vi "Get Item by key.vi"(8 "error in (no error)":errorcluster caption="错误输入（无错误）", 10 "Key":variant, 11 "HashTable 输入":refnum<class "HashTable.lvclass"> caption="DNL_LabVIEW Object in") -> (0 "error out":errorcluster caption="错误输出", 2 "Value":variant, 3 "HashTable 输出":refnum<class "HashTable.lvclass"> caption="DNL_LabVIEW Object out")   [LabVIEW 2012, in "HashTable.lvclass"]
uses:
  HashTable.lvclass
  HashTable.lvclass/HashTable.ctl
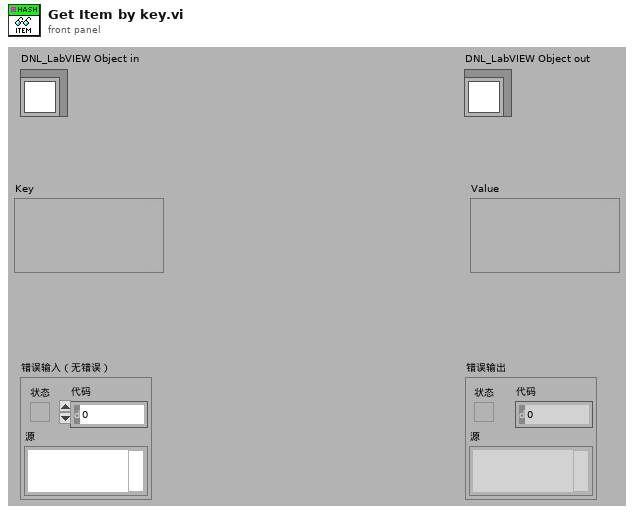
[diagram p1: front panel]
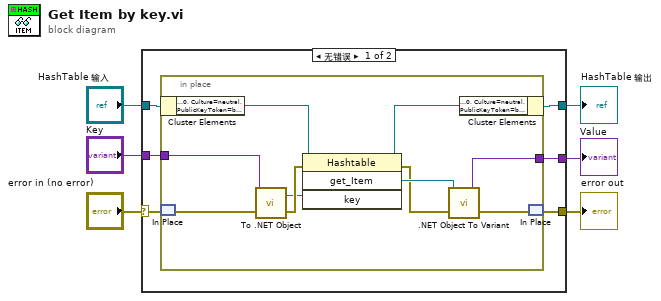
[diagram p0: block diagram]
diagram:
  n1 = case shown="无错误" "error in (no error)" {
    selector: "error in (no error)" -> [w10 w24]
    tunnel: [w7 w24] -> w5
    tunnel: [w11 w23] -> w3
    tunnel: "HashTable 输入" -> [w12 w23]
    tunnel: "Key" -> [w9 _]
    tunnel: [w8 _] -> w1
    frame No Error {
      n2 = in-place {
        in-place-border: w9 -> [w18]
        in-place-border: [w15] -> w8
        n3 = in-place-cluster #1(w12) -> ("HashTable"=w22:refnum<k24>)
        n4 = in-place-match #2(w10) -> (w20:errorcluster)
        n5 = call <vilib>:"To .NET Object.vi"("error in (no error)"=w20, "anything"=w18) -> ("error out"=w19:errorcluster, ".NET object"=w13:refnum<k24>)
        n6 = invoke class="Hashtable" method="get_Item"(reference=w22, error in=w19, "key"=w13) -> (reference out=w21:refnum<k24>, error out=w16:errorcluster, "get_Item"=w17:refnum<k24>)  [unwired: 1 in, 1 out]
        n7 = call <vilib>:".NET Object To Variant.vi"("error in (no error)"=w16, ".NET object"=w17) -> ("error out"=w14:errorcluster, "variant"=w15:variant)
        n8 = in-place-cluster #1("HashTable"=w21) -> (w11:refnum<class "HashTable.lvclass">)
        n9 = in-place-match #2(w14) -> (w7:errorcluster)
      }
    }
    frame Error {
    }
  }
  "error out" <- w5
  "HashTable 输出" <- w3
  "Value" <- w1
